vi "acqWaveform.vi"(0 "OSC in":refnum<visa-resource-name>, 1 "Points":u32=5000 max=7000, 2 "error in (no error)":errorcluster) -> (3 "OSC out":refnum<visa-resource-name>, 4 "time sequence":dbl[](array[numeric]), 5 "Voltage sequence":dbl[](array[numeric]), 6 "error out":errorcluster)   [LabVIEW 2016]
panel:
  out "XY Graph":cluster{dbl[], dbl[]}(graph)
  out "String":string
  in  "Channel":i8=1
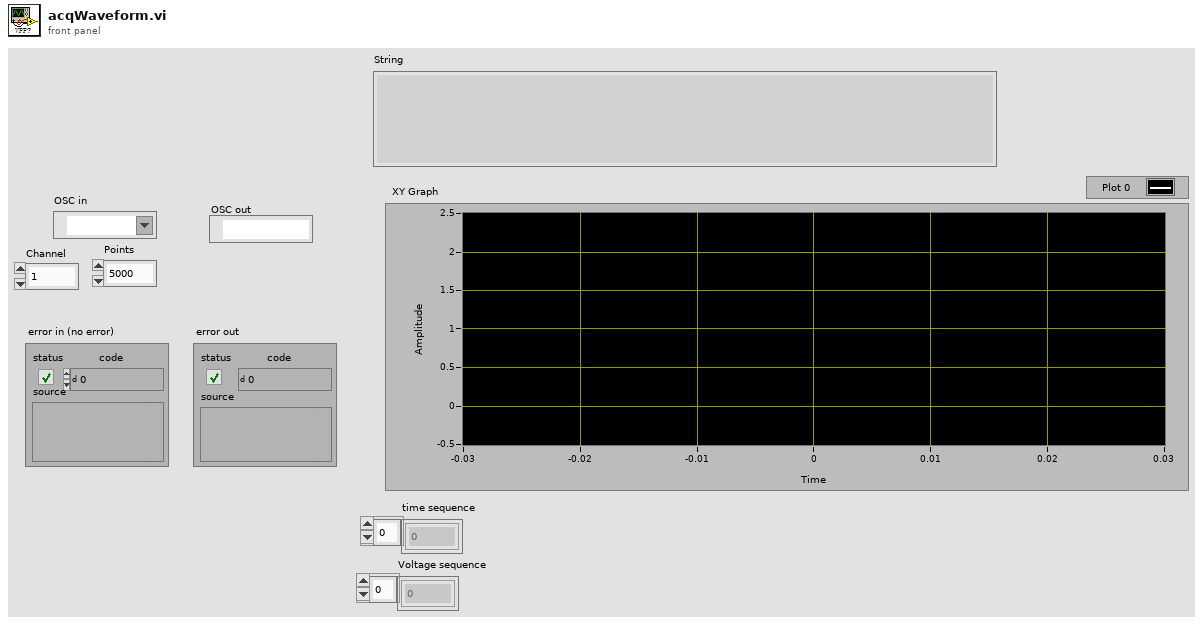
[diagram p1: front panel]
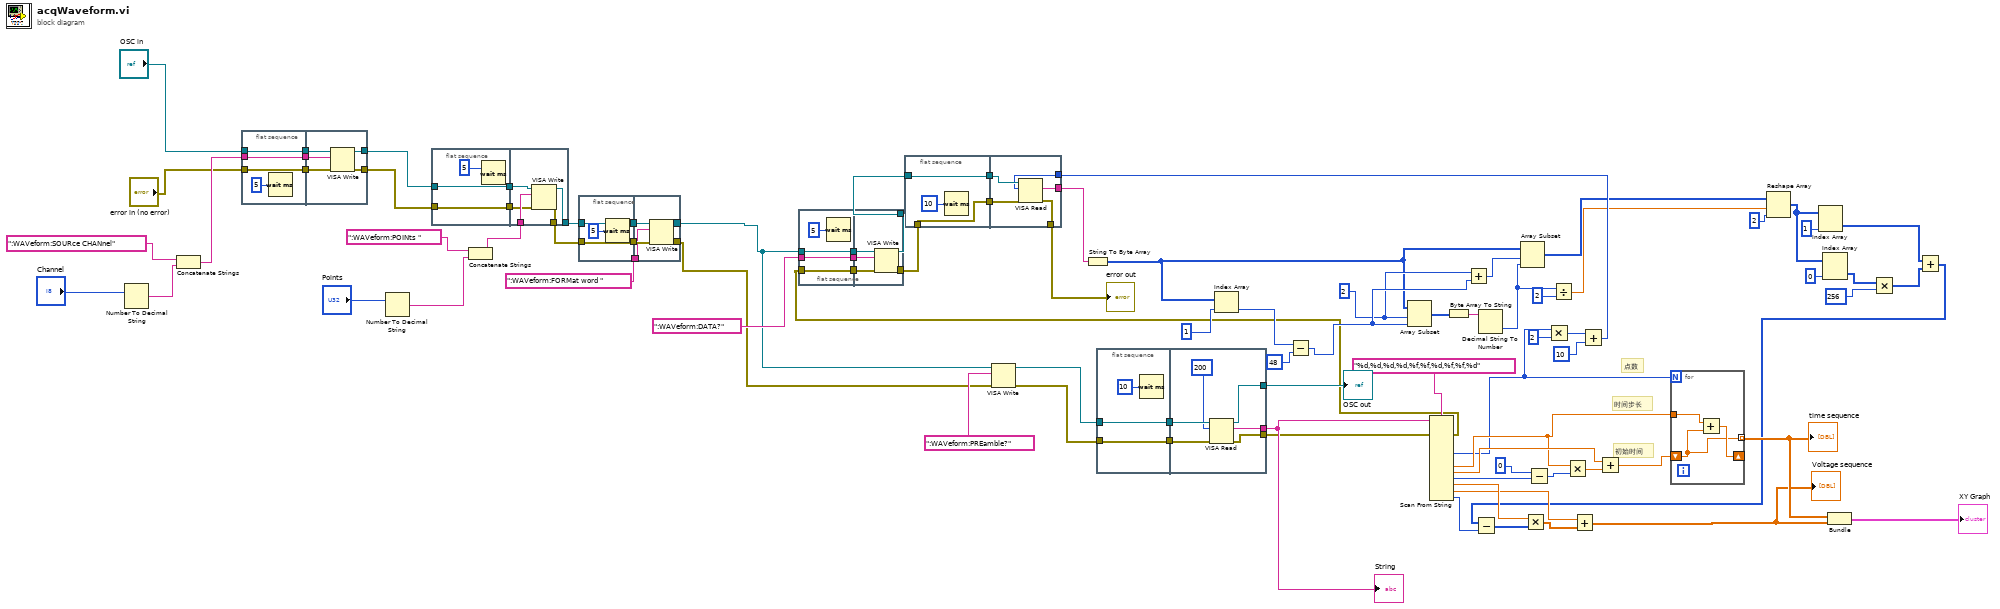
[diagram p0: block diagram]
diagram:
  w66 = 2
  # "初始时间"
  # "时间步长"
  # "点数"
  n1 = Number To Decimal String(number="Channel") -> (decimal integer string=w84:string)  [unwired: 1 in]
  n2 = Concatenate Strings(":WAVeform:SOURce CHANnel", w84) -> (w83:string)
  n3 = flat-sequence {
    tunnel: "error in (no error)" -> [w88]
    tunnel: "OSC in" -> [w89]
    tunnel: w83 -> [w90]
    tunnel: [w90] -> w32
    tunnel: [w89] -> w31
    tunnel: [w88] -> w30
    tunnel: [w94] -> w79
    tunnel: [w93] -> w78
    tunnel: w32 -> [w95]
    tunnel: w31 -> [w92]
    tunnel: w30 -> [w91]
    frame #0 {
      n4 = Wait (ms)(milliseconds to wait=u32 5) -> ()  [unwired: 1 out]
    }
    frame #1 {
      n5 = VISA Write(VISA resource name=w92, write buffer=w95, error in (no error)=w91) -> (VISA resource name out=w93:refnum<visa-resource-name>, error out=w94:errorcluster)  [unwired: 1 out]
    }
  }
  n6 = Number To Decimal String(number="Points") -> (decimal integer string=w82:string)  [unwired: 1 in]
  n7 = flat-sequence {
    tunnel: w78 -> [w97]
    tunnel: w79 -> [w98]
    tunnel: [w98] -> w29
    tunnel: [w97] -> w28
    tunnel: w80 -> [w103]
    tunnel: [w100] -> w77
    tunnel: [w99] -> w76
    tunnel: w29 -> [w102]
    tunnel: w28 -> [w101]
    frame #0 {
      n8 = Wait (ms)(milliseconds to wait=u32 5) -> ()  [unwired: 1 out]
    }
    frame #1 {
      n9 = VISA Write(VISA resource name=w101, write buffer=w103, error in (no error)=w102) -> (VISA resource name out=w100:refnum<visa-resource-name>, error out=w99:errorcluster)  [unwired: 1 out]
    }
  }
  n10 = Concatenate Strings(":WAVeform:POINts ", w82) -> (w80:string)
  n11 = flat-sequence {
    tunnel: w76 -> [w105]
    tunnel: w77 -> [w106]
    tunnel: [w106] -> w27
    tunnel: [w105] -> w26
    tunnel: ":WAVeform:FORMat word " -> [w109]
    tunnel: w27 -> [w111]
    tunnel: w26 -> [w110]
    tunnel: [w108] -> w16
    tunnel: [w107] -> w22
    frame #0 {
      n12 = Wait (ms)(milliseconds to wait=u32 5) -> ()  [unwired: 1 out]
    }
    frame #1 {
      n13 = VISA Write(VISA resource name=w111, write buffer=w109, error in (no error)=w110) -> (VISA resource name out=w108:refnum<visa-resource-name>, error out=w107:errorcluster)  [unwired: 1 out]
    }
  }
  n14 = flat-sequence {
    tunnel: w10 -> [w113]
    tunnel: w16 -> [w114]
    tunnel: ":WAVeform:DATA?" -> [w115]
    tunnel: [w115] -> w25
    tunnel: [w114] -> w24
    tunnel: [w113] -> w23
    tunnel: [w117] -> w41
    tunnel: [w116] -> w39
    tunnel: w25 -> [w120]
    tunnel: w24 -> [w119]
    tunnel: w23 -> [w118]
    frame #0 {
      n15 = Wait (ms)(milliseconds to wait=u32 5) -> ()  [unwired: 1 out]
    }
    frame #1 {
      n16 = VISA Write(VISA resource name=w119, write buffer=w120, error in (no error)=w118) -> (VISA resource name out=w117:refnum<visa-resource-name>, error out=w116:errorcluster)  [unwired: 1 out]
    }
  }
  n17 = flat-sequence {
    tunnel: w41 -> [w122]
    tunnel: [w122] -> w40
    tunnel: w39 -> [w121]
    tunnel: [w121] -> w38
    tunnel: w40 -> [w125]
    tunnel: w38 -> [w126]
    tunnel: [w128] -> w37
    tunnel: [w127] -> w21
    tunnel: w15 -> [w124]
    frame #0 {
      n18 = Wait (ms)(milliseconds to wait=u32 10) -> ()  [unwired: 1 out]
    }
    frame #1 {
      n19 = VISA Read(VISA resource name=w125, byte count=w124, error in (no error)=w126) -> (read buffer=w128:string, error out=w127:errorcluster)  [unwired: 2 out]
    }
  }
  n20 = VISA Write(VISA resource name=w16, write buffer=":WAVeform:PREamble?", error in (no error)=w22) -> (VISA resource name out=w62:refnum<visa-resource-name>, error out=w61:errorcluster)  [unwired: 1 out]
  n21 = String To Byte Array(string=w37) -> (unsigned byte array=w64:u8[])
  n22 = flat-sequence {
    tunnel: w61 -> [w130]
    tunnel: w62 -> [w131]
    tunnel: [w131] -> w36
    tunnel: [w130] -> w35
    tunnel: [w135] -> w60
    tunnel: [w133] -> w58
    tunnel: [w132] -> w57
    tunnel: w36 -> [w137]
    tunnel: w35 -> [w136]
    frame #0 {
      n23 = Wait (ms)(milliseconds to wait=u32 10) -> ()  [unwired: 1 out]
    }
    frame #1 {
      n24 = VISA Read(VISA resource name=w137, byte count=200, error in (no error)=w136) -> (VISA resource name out=w135:refnum<visa-resource-name>, read buffer=w133:string, error out=w132:errorcluster)  [unwired: 1 out]
    }
  }
  n25 = Index Array(array=w64, index=1) -> (element=w71:u8)
  n26 = Subtract(x=w71, y=48) -> (x-y=w67:i32)
  n27 = Array Subset(array=w64, index=w66, length=w67) -> (w69:u8[])
  n28 = Scan From String(format string="%d,%d,%d,%d,%f,%f,%d,%f,%f,%d", input string=w58, error in=w57) -> (error out=w10:errorcluster, output 3=w20:i32, output 5=w50:dbl, output 6=w52:dbl, output 7=w56:i32, output 8=w47:dbl, output 9=w46:dbl, output 10=w49:i32)  [unwired: 14 in, 2 out]
  n29 = Byte Array To String(unsigned byte array=w69) -> (string=w68:string)
  n30 = Add(x=w66, y=w67) -> (x+y=w65:i32)
  n31 = Decimal String To Number(string=w68) -> (number=w13:i32)  [unwired: 2 in, 1 out]
  n32 = Array Subset(array=w64, index=w65, length=w13) -> (w3:u8[])
  n33 = Subtract(x=0, y=w56) -> (x-y=w54:i32)
  n34 = Multiply(x=w20, y=2) -> (x*y=w18:i32)
  n35 = Divide(x=w13, y=2) -> (x/y=w11:dbl)
  n36 = Multiply(x=w50, y=w54) -> (x*y=w53:dbl)
  n37 = Add(x=w18, y=10) -> (x+y=w15:i32)
  n38 = Add(x=w52, y=w53) -> (x+y=w51:dbl)
  n39 = for {
    N: w20 -> [_]
    shift-right: [w140] -> _
    shift-left: w51 -> [w138]
    tunnel: w50 -> [w139]
    tunnel: [w138] -> w44 mode=indexing
    n40 = Add(x=w139, y=w138) -> (x+y=w140:dbl)
  }
  "time sequence" <- w44
  n41 = Reshape Array(w3, w11, 2 ("dimension size")) -> (w9:u8[][])
  n42 = Index Array(array=w9, index (col)=1 ("disabled index (col)")) -> (element=w5:u8[])  [unwired: 1 in]
  n43 = Index Array(array=w9, index (col)=0 ("disabled index (col)")) -> (element=w7:u8[])  [unwired: 1 in]
  n44 = Multiply(x=w7, y=256) -> (x*y=w4:i32[])
  n45 = Add(x=w5, y=w4) -> (x+y=w2:i32[])
  n46 = Subtract(x=w2, y=w49) -> (x-y=w48:i32[])
  n47 = Multiply(x=w47, y=w48) -> (x*y=w45:dbl[])
  n48 = Add(x=w46, y=w45) -> (x+y=w42:dbl[])
  "Voltage sequence" <- w42
  n49 = Bundle(w44, w42) -> (→"XY Graph":cluster{dbl[], dbl[]})  [unwired: 1 in]
  "OSC out" <- w60
  "error out" <- w21
  "String" <- w58
